vi "tdm_write.vi"() -> ()   [LabVIEW 2019]
panel:
  in  "Noise amplitude":dbl=0.6
  out "Waveform Graph":dynamicdata(graph)
  in  "Knob":dbl(knob) scale=0.0..10.0
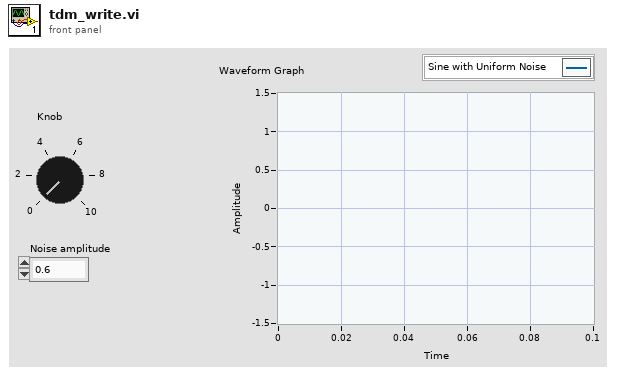
[diagram p1: front panel]
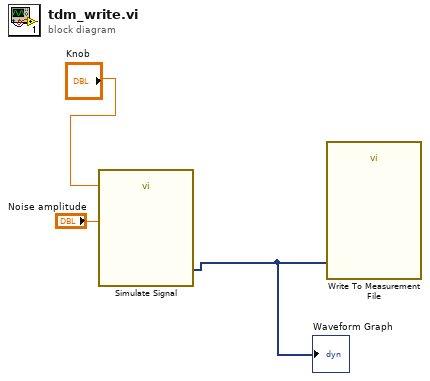
[diagram p0: block diagram]
diagram:
  n1 = call "Simulate Signal"("Frequency"="Knob", "Noise amplitude"="Noise amplitude") -> ("Sine with Uniform Noise"=w3:dynamicdata)  [unwired: 12 in, 1 out]
  "Waveform Graph" <- w3
  n2 = call "Write To Measurement File"("Signals"=w3) -> ()  [unwired: 16 in, 3 out]
